vi "Data Loop.vi"(0 "Waveform Data":dbl[](array[numeric]), 1 "Samples Per Average":i32, 7 "Data Array in":dbl[][](array[numeric]), 9 "Reset?":bool, 13 "Voltage to AU Conversion Factor":dbl) -> (4 "XY out":cluster{"X":dbl, "Y":dbl}[](array[cluster]), 8 "Data Array out":dbl[][](array[numeric]))   [LabVIEW 2016]
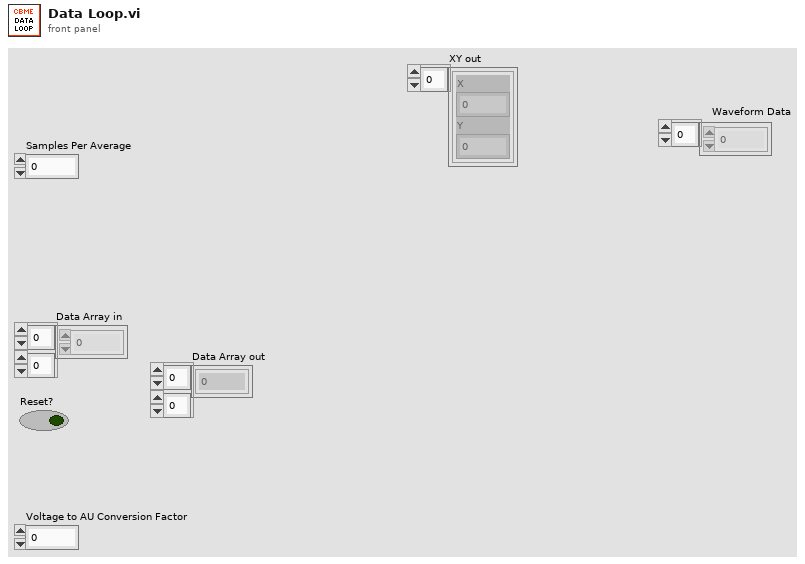
[diagram p1: front panel]
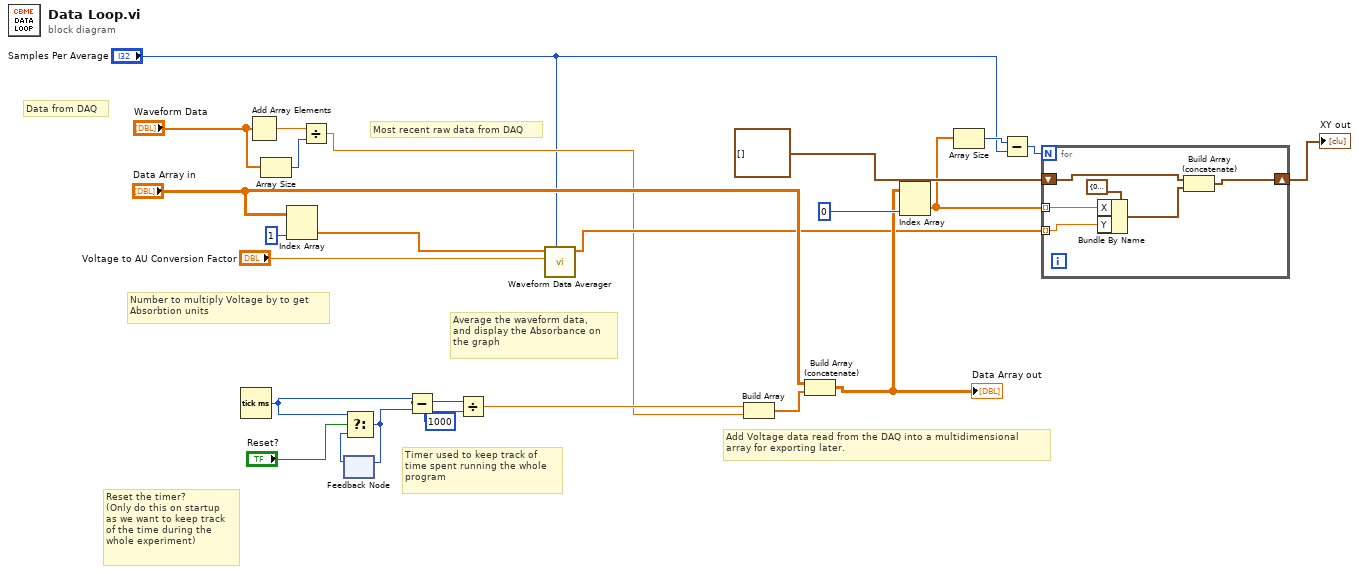
[diagram p0: block diagram]
diagram:
  # "Average the waveform data,\nand display the Absorbance on\nthe graph"
  # "Most recent raw data from DAQ"
  # "Reset the timer?\n(Only do this on startup\nas we want to keep track \nof the time during the \nwhole experiment)"
  # "Number to multiply Voltage by to get\nAbsorbtion units"
  # "Data from DAQ"
  # "Add Voltage data read from the DAQ into a multidimensional\narray for exporting later."
  # "Timer used to keep track of\ntime spent running the whole\nprogram"
  n1 = Tick Count (ms)() -> (millisecond timer value=w22:u32)
  n2 = Add Array Elements(numeric array="Waveform Data") -> (sum=w16:dbl)
  n3 = Array Size(array="Waveform Data") -> (size(s)=w15:i32)
  n4 = Index Array(array="Data Array in", index (col)=1 ("disabled index (col)")) -> (element=w7:dbl[])  [unwired: 1 in]
  n5 = Divide(x=w16, y=w15) -> (x/y=w5:dbl)
  n6 = feedback #1() -> (w20:u32)  [unwired: 1 in]
  n7 = Select(t=w22, s="Reset?", f=w20) -> (s? t:f=w19:u32)
  n8 = feedback-in #1(w19) -> ()
  n9 = Subtract(x=w22, y=w19) -> (x-y=w23:u32)
  n10 = Divide(x=w23, y=u32 1000) -> (x/y=w25:dbl)
  n11 = call "Waveform Data Averager.vi"("Samples Per Average"="Samples Per Average", "V to AU Conversion"="Voltage to AU Conversion Factor", "Voltage Array In"=w7) -> ("Voltage Array Out"=w6:dbl[])  [unwired: 7 in, 1 out]
  n12 = Build Array(w25, w5) -> (w18:dbl[])
  n13 = Build Array (concatenate)("Data Array in", w18) -> (w9:dbl[][])
  "Data Array out" <- w9
  n14 = Index Array(array=w9, index (col)=0 ("disabled index (col)")) -> (element=w4:dbl[])  [unwired: 1 in]
  n15 = Array Size(array=w4) -> (size(s)=w3:i32)
  n16 = Subtract(x=w3, y="Samples Per Average") -> (x-y=w1:i32)
  n17 = for {
    N: w1 -> [_]
    tunnel: w6 -> [w29] mode=indexing
    shift-right: [w26] -> w8
    shift-left: cluster{"X":dbl, "Y":dbl}[] [] -> [w28]
    tunnel: w4 -> [w30] mode=indexing
    n18 = Bundle By Name(cluster=cluster{"X":dbl, "Y":dbl} {"X"=0.0, "Y"=0.0}, "X"=w30, "Y"=w29) -> (w27:cluster{"X":dbl, "Y":dbl})
    n19 = Build Array (concatenate)(w28, w27) -> (w26:cluster{"X":dbl, "Y":dbl}[])
  }
  "XY out" <- w8
